vi "dlgMultiAnalysisList.vi"(7 "StandAlone (true)":bool=TRUE, 8 "error in (no error)":errorcluster) -> (0 "error out":errorcluster, 1 "Analyse":bool, 3 "FileList":string[][](array[string]))   [LabVIEW 2014]
uses:
  typedefs/eMainAction.ctl
  <vilib>/Utility/miscctls.llb/LVRowAndColumnTypeDef.ctl
  typedefs/ePathsAction.ctl
  <vilib>/Utility/file.llb/Read From Spreadsheet File (string).vi
  <vilib>/Utility/file.llb/Write To Spreadsheet File (string).vi
panel:
  in  "btnPopulate":bool
  in  "btnDelete":bool
  in  "btnClear":bool
  in  "btnInsert":bool
  in  "btnAnalyse":bool
  in  "btnCancel":bool
  in  "lstFiles":string[][](table) caption="List of Files to Analyse"
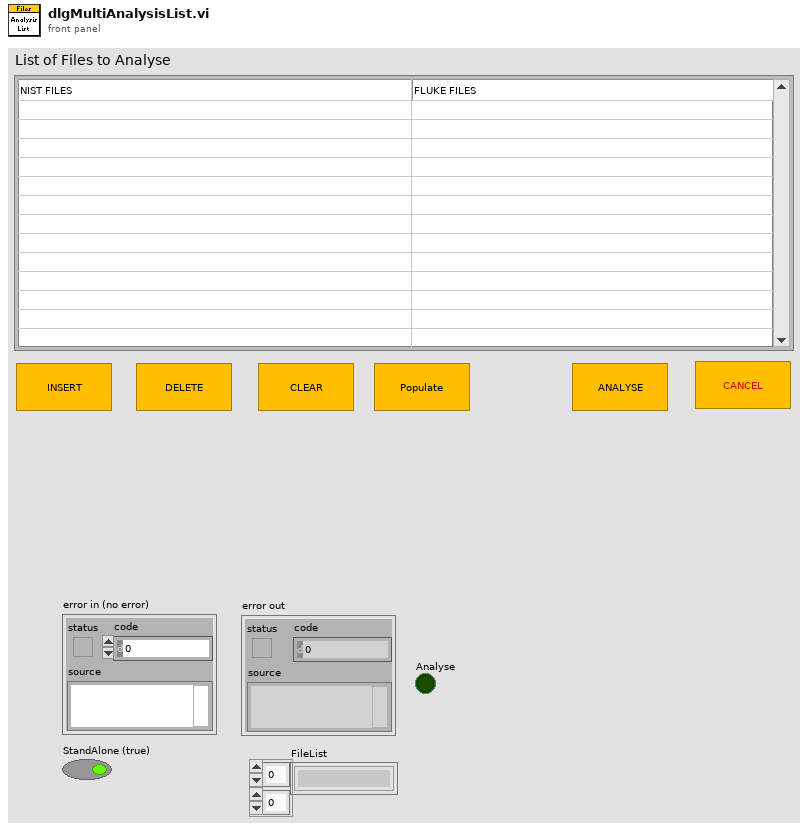
[diagram p1: front panel]
types:
  T1 = typedef "LVRowAndColumnTypeDef.ctl" = cluster{"Row":i32, "Column":i32}
  T2 = typedef "eMainAction.ctl" = enum16{"Init", "ProcessUI", "Exit"}
  T3 = typedef "ePathsAction.ctl" = enum16{"Set", "Get", "Load", "Save", "Default", "Exit"}
  T4 = typedef "Paths.ctl" = cluster{"BasePath":path, "CutPath":path, "LastCutPath":path, "CCSPath":path, "LastCCSPath":path, "ResultsPath":path}
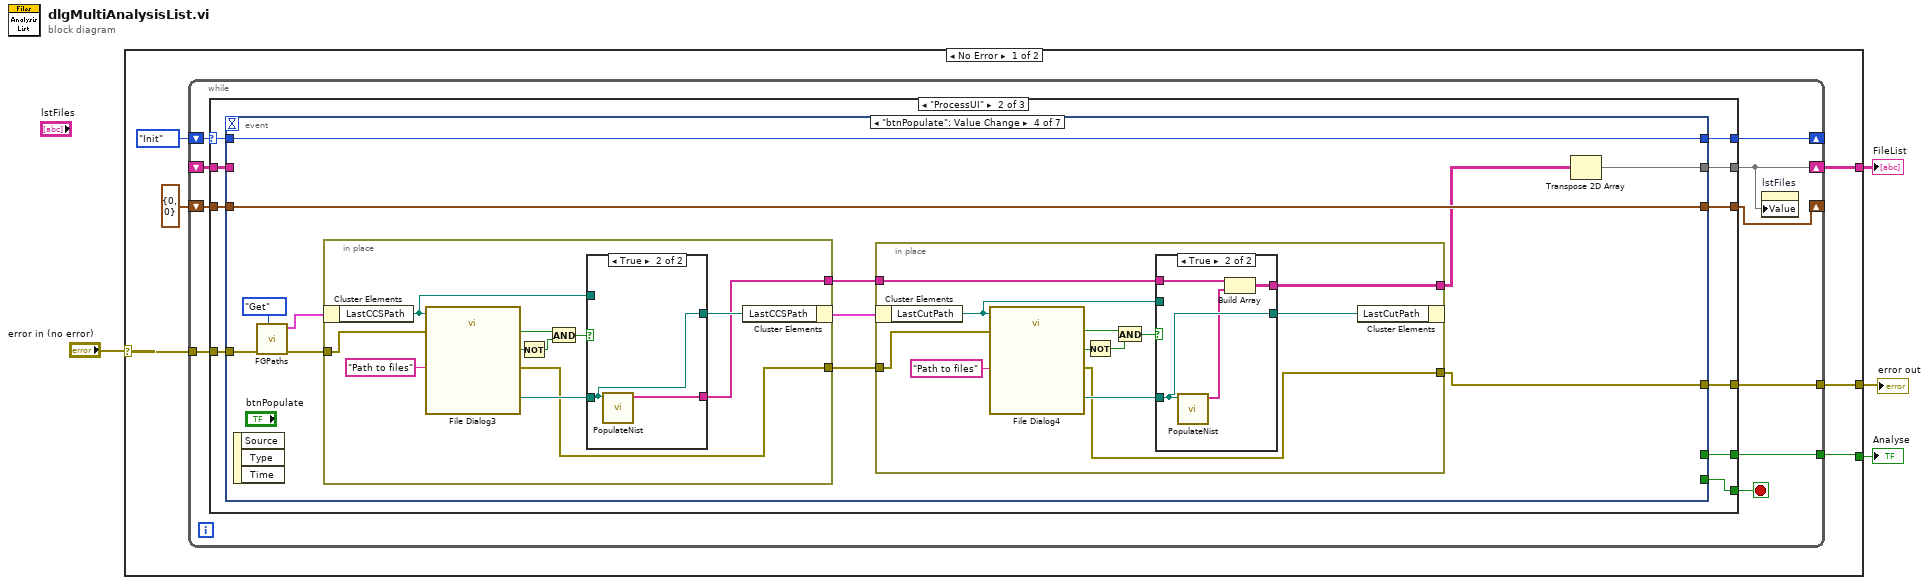
[diagram p0: block diagram]
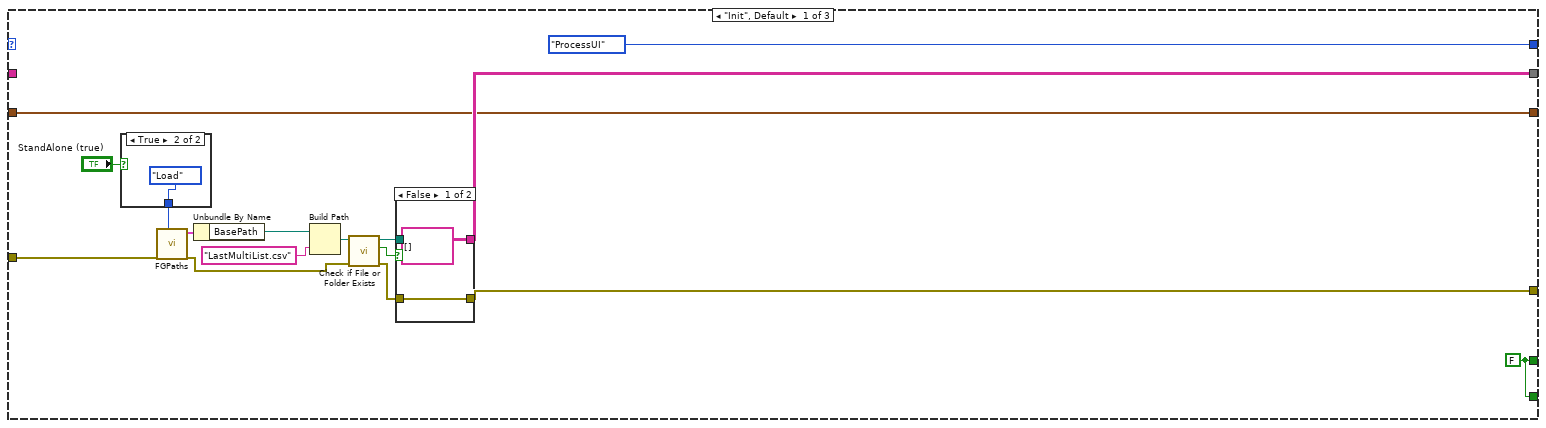
[diagram p2: hidden frame]
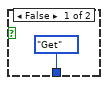
[diagram p3: hidden frame]
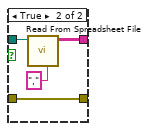
[diagram p4: hidden frame]
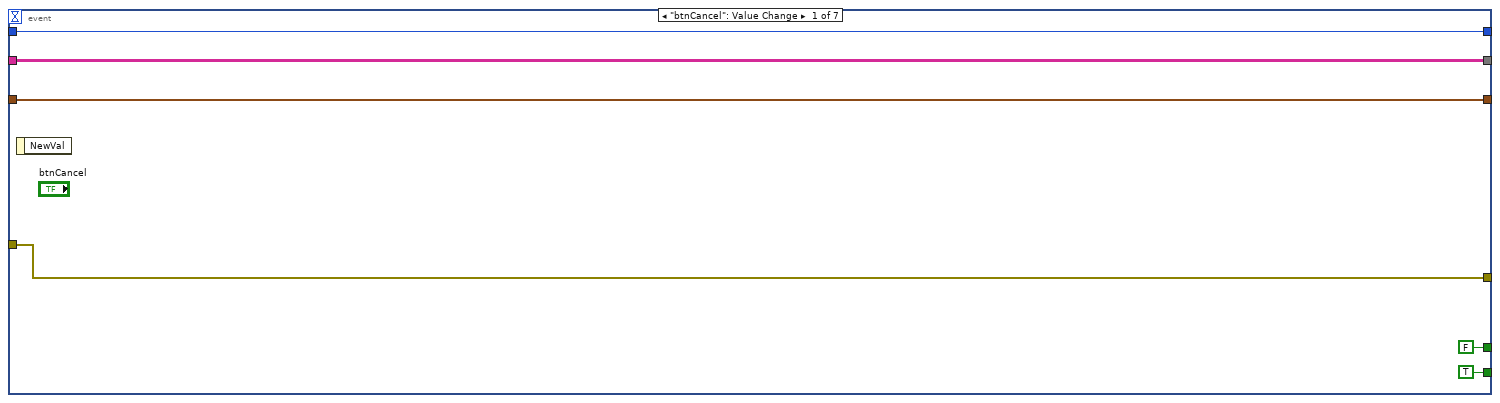
[diagram p5: hidden frame]
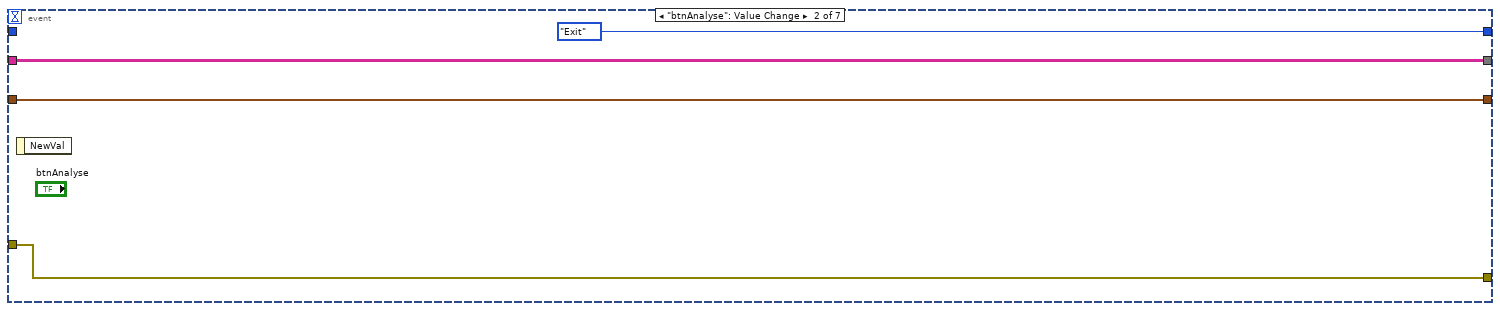
[diagram p6: hidden frame]
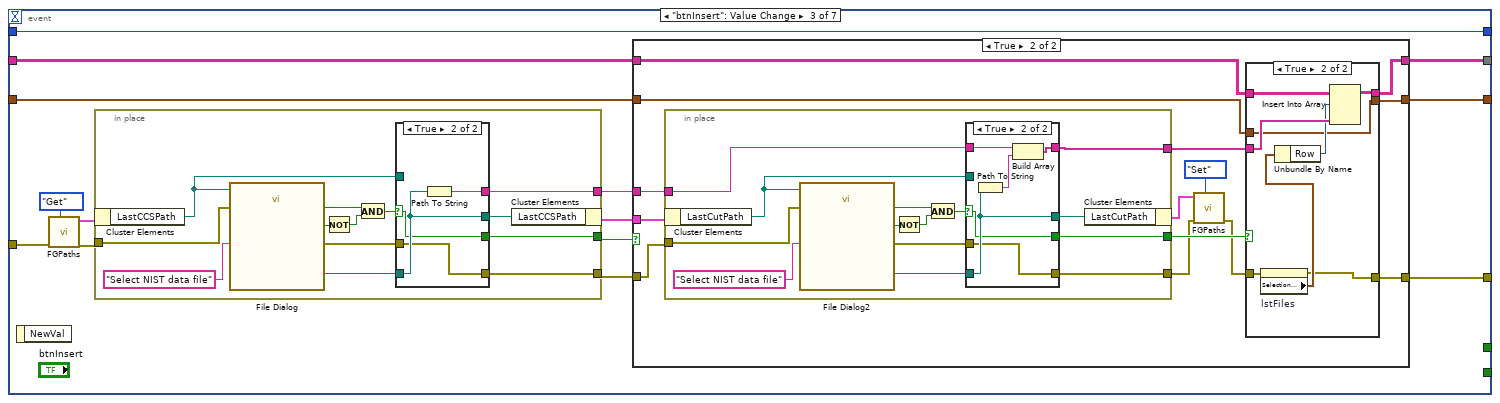
[diagram p7: hidden frame]
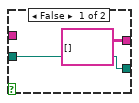
[diagram p12: hidden frame]
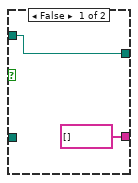
[diagram p13: hidden frame]
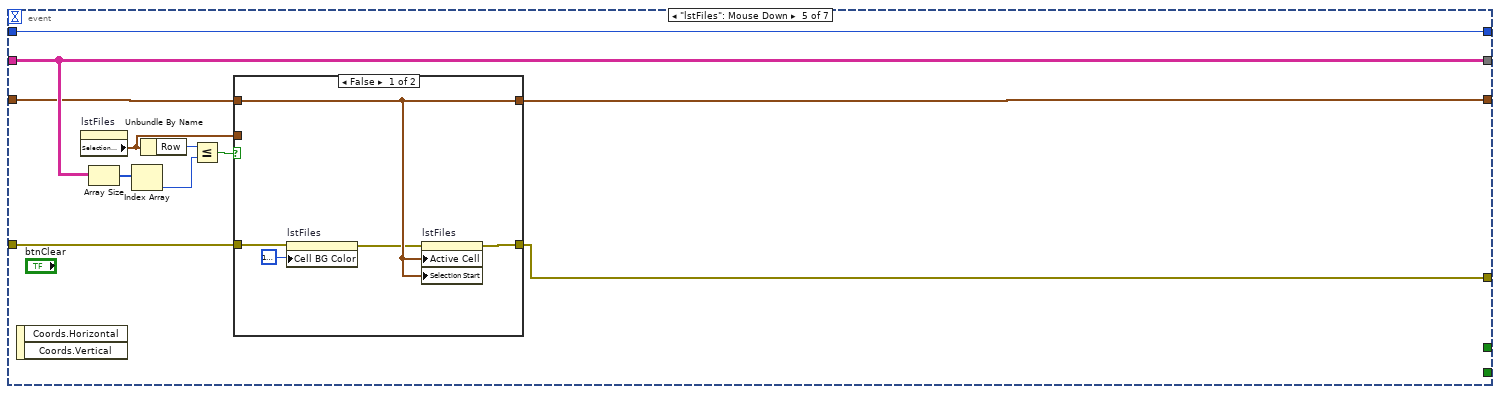
[diagram p14: hidden frame]
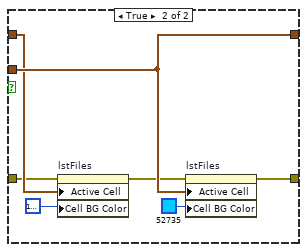
[diagram p15: hidden frame]
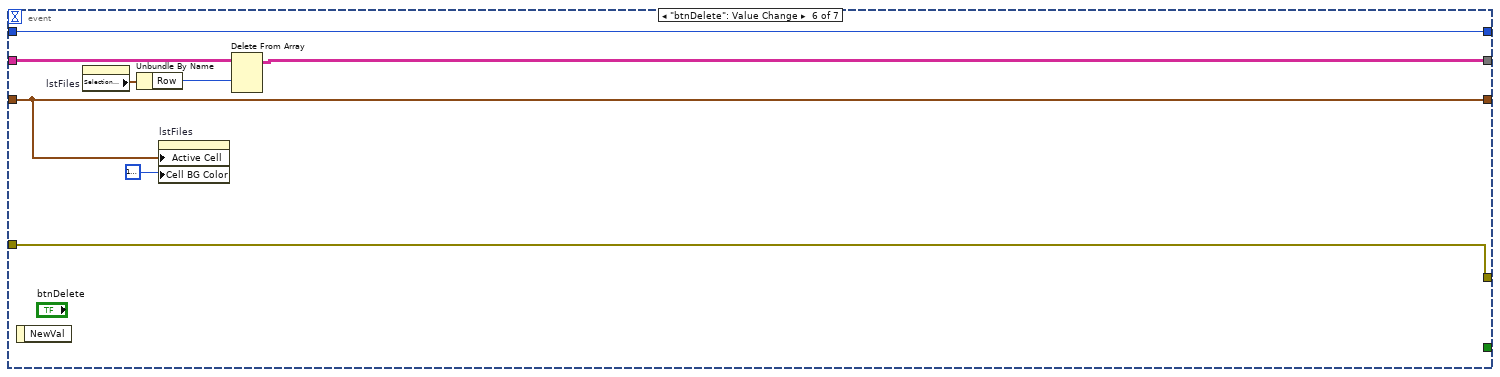
[diagram p16: hidden frame]
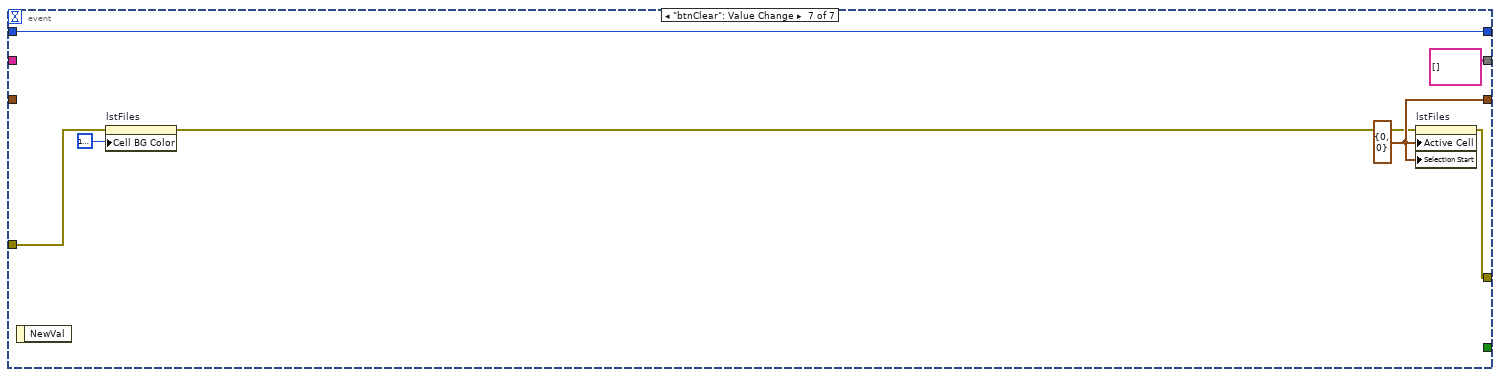
[diagram p17: hidden frame]
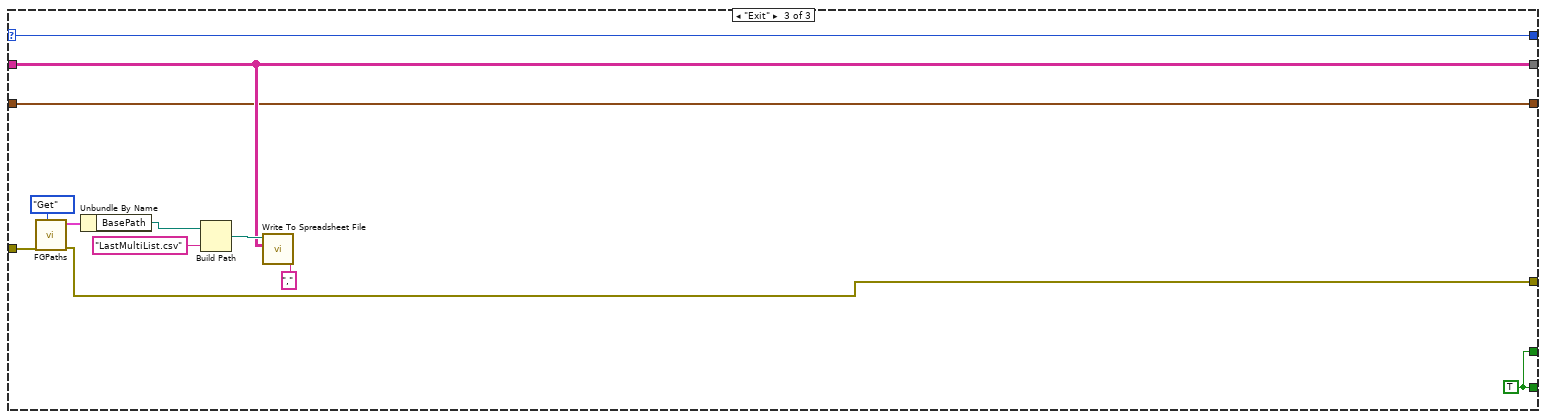
[diagram p18: hidden frame]
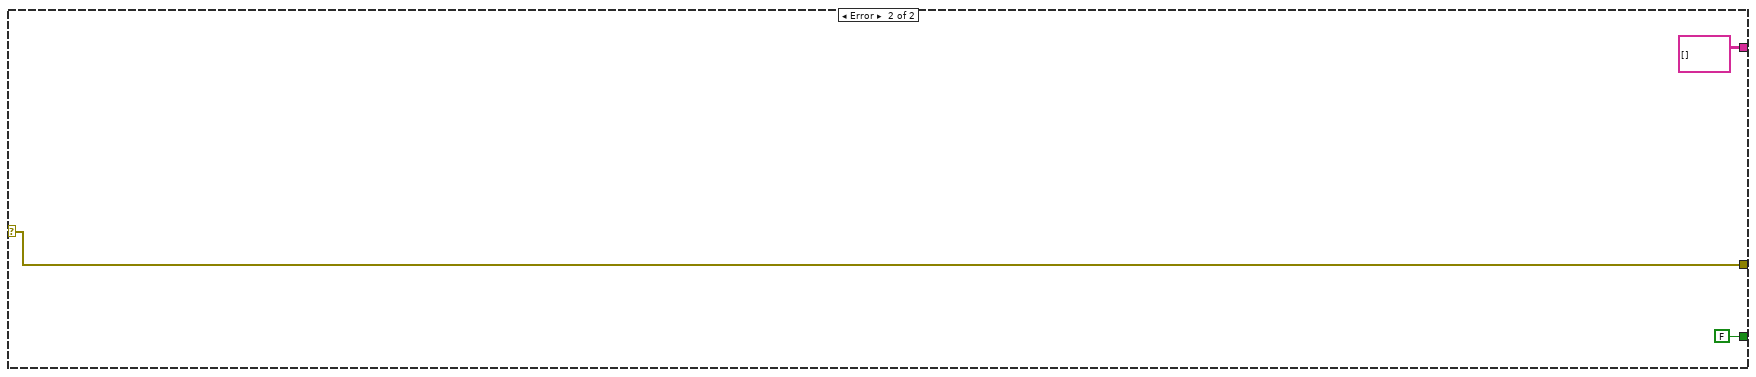
[diagram p19: hidden frame]
diagram:
  n1 = case shown="No Error" "error in (no error)" {
    selector: "error in (no error)" -> [w10 w245]
    tunnel: [w8 FALSE] -> w3
    tunnel: [w7 string[][] [] ("all rows")] -> w2
    tunnel: [w5 w245] -> w1
    frame No Error {
      n2 = while {
        tunnel: w10 -> [w20]
        shift-right: [w17] -> _
        shift-left: eMainAction."Init" ("eMainAction") -> [w19]
        shift-right: [w18] -> w7
        shift-left: _ -> [w14]
        tunnel: [w15] -> w8
        shift-right: [w13] -> _
        shift-left: T1 {"Row"=0, "Column"=0} ("Selection Start") -> [w12]
        tunnel: [w11] -> w5
        stop <- w16 stop-if-true
        n3 = case shown="\"ProcessUI\"" w19 {
          selector: w19 -> [_ w51 w235]
          tunnel: w20 -> [w26 w48 w243]
          tunnel: [w25 w50 w236] -> w18
          tunnel: [eMainAction."ProcessUI" ("eMainAction") w52 w235] -> w17
          tunnel: [w23 w54 w244] -> w16
          tunnel: [w23 w53 w244] -> w15
          tunnel: w14 -> [_ w49 w236]
          tunnel: [w22 w47 w234] -> w13
          tunnel: w12 -> [w22 w46 w234]
          tunnel: [w21 w45 w233] -> w11
          frame "Init", Default {
            w23 = FALSE
            n4 = case shown="True" "StandAlone (true)" {
              tunnel: [ePathsAction."Get" ("ePathsAction") ePathsAction."Load" ("ePathsAction")] -> w36
              frame False {
              }
              frame True {
              }
            }
            n5 = call "FGPaths.vi"("ePathsAction"=w36, "error in (no error)"=w26) -> ("error out"=w31:errorcluster, "PathsOut"=w35:T4)  [unwired: 8 in]
            n6 = Unbundle By Name(w35) -> ("BasePath"=w34:path)
            n7 = Build Path(base path=w34, name or relative path="LastMultiList.csv") -> (appended path=w32:path)
            n8 = call <vilib>:"Check if File or Folder Exists.vi"("error in (no error)"=w31, "path"=w32) -> ("error out"=w28:errorcluster, "file or folder exists?"=w29:bool, "dup path"=w30:path)  [unwired: 7 in]
            n9 = case shown="False" w29 {
              tunnel: w30 -> [_ w44]
              tunnel: w28 -> [w39 w42]
              tunnel: [w39 w42] -> w21
              tunnel: [string[][] [] ("all rows") w41] -> w25
              frame False {
              }
              frame True {
                n10 = call-poly <vilib>:"Read From Spreadsheet File.vi"("delimiter (\\t)"="," ("delimiter (\\t)"), "file path (dialog if empty)"=w44) -> ("all rows"=w41:string[][])  [unwired: 5 in, 4 out]
              }
            }
          }
          frame "ProcessUI" {
            n11 = event shown="[3] \"btnPopulate\": Value Change" {
              selector: _ -> [_ _ _ _ _ _ _]
              dyn-events: _ -> [_ _ _ _ _ _ _]
              timeout: _ -> [_ _ _ _ _ _ _]
              tunnel: [TRUE _ _ _ _ _ _] -> w54
              tunnel: [FALSE _ _ _ _ _ _] -> w53
              tunnel: [w58 eMainAction."Exit" ("eMainAction") w68 w156 w196 w220 w232] -> w52
              tunnel: w51 -> [w58 _ w68 w156 w196 w220 w232]
              tunnel: [w57 w63 w72 w155 w204 w222 string[][] [] ("all rows")] -> w50
              tunnel: w49 -> [w57 w63 w73 _ w204 w225 _]
              tunnel: w48 -> [w55 w62 w78 w161 w197 w218 w228]
              tunnel: [w56 w61 w65 w157 w199 w219 w230] -> w47
              tunnel: w46 -> [w56 w61 w66 w157 w198 w219 _]
              tunnel: [w55 w62 w67 w150 w195 w218 w226] -> w45
              event "btnCancel": Value Change {
                n12 = event-data() -> ()  [unwired: 1 in, 1 out]
              }
              event "btnAnalyse": Value Change {
                n13 = event-data() -> ()  [unwired: 1 in, 1 out]
              }
              event "btnInsert": Value Change {
                n14 = event-data() -> ()  [unwired: 1 in, 1 out]
                n15 = call "FGPaths.vi"("ePathsAction"=ePathsAction."Get", "error in (no error)"=w78) -> ("error out"=w75:errorcluster, "PathsOut"=w76:T4)  [unwired: 8 in]
                n16 = in-place {
                  in-place-border: w75 -> [w141]
                  in-place-border: [w133] -> w74
                  in-place-border: [w132] -> w69
                  in-place-border: [w130] -> w71
                  n17 = in-place-cluster #1(w76) -> ("LastCCSPath"=w136:path)
                  n18 = call "File Dialog"("start path"=w136, "prompt"="Select NIST data file", "error in"=w141) -> ("selected path"=w134:path, "exists"=w138:bool, "cancelled"=w139:bool, "error out"=w131:errorcluster)  [unwired: 9 in]
                  n19 = Not(x=w139) -> (.not. x?=w137:bool)
                  n20 = And(x=w138, y=w137) -> (x .and. y?=w140:bool)
                  n21 = case shown="True" w140 {
                    selector: w140 -> [w144 w148]
                    tunnel: w136 -> [w145 _]
                    tunnel: [w145 w149] -> w135
                    tunnel: w134 -> [_ w149]
                    tunnel: [_ w146] -> w132
                    tunnel: [w144 w148] -> w133
                    tunnel: w131 -> [w143 w147]
                    tunnel: [w143 w147] -> w130
                    frame False {
                    }
                    frame True {
                      n22 = Path To String(path=w149) -> (string=w146:string)
                    }
                  }
                  n23 = in-place-cluster #1("LastCCSPath"=w135) -> (w70:T4)
                }
                n24 = case shown="True" w74 {
                  tunnel: w73 -> [w81 w92]
                  tunnel: [w81 w91] -> w72
                  tunnel: w71 -> [w80 w94]
                  tunnel: w70 -> [_ w95]
                  tunnel: [w80 w88] -> w67
                  tunnel: w69 -> [_ w90]
                  tunnel: w66 -> [w79 w86]
                  tunnel: [w79 w87] -> w65
                  frame False {
                  }
                  frame True {
                    n25 = in-place {
                      in-place-border: w94 -> [w119]
                      in-place-border: [w111] -> w93
                      in-place-border: [w109] -> w83
                      in-place-border: w90 -> [w108]
                      in-place-border: [w107] -> w89
                      n26 = in-place-cluster #2(w95) -> ("LastCutPath"=w114:path)
                      n27 = call "File Dialog2"("start path"=w114, "prompt"="Select NIST data file", "error in"=w119) -> ("selected path"=w112:path, "exists"=w116:bool, "cancelled"=w117:bool, "error out"=w110:errorcluster)  [unwired: 9 in]
                      n28 = Not(x=w117) -> (.not. x?=w115:bool)
                      n29 = And(x=w116, y=w115) -> (x .and. y?=w118:bool)
                      n30 = case shown="True" w118 {
                        selector: w118 -> [w122 w128]
                        tunnel: w114 -> [w123 _]
                        tunnel: [w123 w129] -> w113
                        tunnel: w112 -> [_ w129]
                        tunnel: [w122 w128] -> w111
                        tunnel: w110 -> [w121 w127]
                        tunnel: [w121 w127] -> w109
                        tunnel: w108 -> [_ w125]
                        tunnel: [_ w126] -> w107
                        frame False {
                        }
                        frame True {
                          n31 = Path To String(path=w129) -> (string=w124:string)
                          n32 = Build Array(w125, w124) -> (w126:string[])
                        }
                      }
                      n33 = in-place-cluster #2("LastCutPath"=w113) -> (w85:T4)
                    }
                    n34 = call "FGPaths.vi"("ePathsAction"=ePathsAction."Set", "error in (no error)"=w83, "PathsIn"=w85) -> ("error out"=w82:errorcluster)  [unwired: 7 in, 1 out]
                    n35 = case shown="True" w93 {
                      tunnel: w92 -> [w98 w106]
                      tunnel: [w98 w105] -> w91
                      tunnel: w89 -> [_ w104]
                      tunnel: w82 -> [w97 w101]
                      tunnel: [w97 w100] -> w88
                      tunnel: [w96 w99] -> w87
                      tunnel: w86 -> [w96 w99]
                      frame False {
                      }
                      frame True {
                        n36 = property on="lstFiles" class="Tbl (strict)"(error in=w101) -> (error out=w100:errorcluster, "Selection Start"=w103:T1)  [unwired: 1 in, 1 out]
                        n37 = Unbundle By Name(w103) -> ("Row"=w102:i32)
                        n38 = Insert Into Array(array=w106, index (row)=w102, new element=w104) -> (w105:string[][])  [unwired: 1 in]
                      }
                    }
                  }
                }
              }
              event "btnPopulate": Value Change {
                n39 = event-data() -> ()  [unwired: 1 in, 3 out]
                n40 = call "FGPaths.vi"("ePathsAction"=ePathsAction."Get", "error in (no error)"=w161) -> ("error out"=w158:errorcluster, "PathsOut"=w159:T4)  [unwired: 8 in]
                n41 = in-place {
                  in-place-border: w158 -> [w189]
                  in-place-border: [w181] -> w154
                  in-place-border: [w180] -> w152
                  n42 = in-place-cluster #3(w159) -> ("LastCCSPath"=w183:path)
                  n43 = call "File Dialog3"("start path"=w183, "prompt"="Path to files", "error in"=w189) -> ("selected path"=w184:path, "exists"=w187:bool, "cancelled"=w188:bool, "error out"=w180:errorcluster)  [unwired: 9 in]
                  n44 = Not(x=w188) -> (.not. x?=w186:bool)
                  n45 = And(x=w187, y=w186) -> (x .and. y?=w185:bool)
                  n46 = case shown="True" w185 {
                    tunnel: w184 -> [_ w193]
                    tunnel: w183 -> [w192 _]
                    tunnel: [w192 w193] -> w182
                    tunnel: [string[] [] ("Array") w194] -> w181
                    frame False {
                    }
                    frame True {
                      n47 = call "PopulateNist.vi"("Path"=w193) -> ("Array"=w194:string[])  [unwired: 10 in]
                    }
                  }
                  n48 = in-place-cluster #3("LastCCSPath"=w182) -> (w153:T4)
                }
                n49 = in-place {
                  in-place-border: w154 -> [w164]
                  in-place-border: w152 -> [w172]
                  in-place-border: [w163] -> w151
                  in-place-border: [w162] -> w150
                  n50 = in-place-cluster #4(w153) -> ("LastCutPath"=w165:path)
                  n51 = call "File Dialog4"("start path"=w165, "prompt"="Path to files", "error in"=w172) -> ("selected path"=w167:path, "exists"=w169:bool, "cancelled"=w171:bool, "error out"=w162:errorcluster)  [unwired: 9 in]
                  n52 = Not(x=w171) -> (.not. x?=w170:bool)
                  n53 = And(x=w169, y=w170) -> (x .and. y?=w168:bool)
                  n54 = case shown="True" w168 {
                    tunnel: w167 -> [_ w179]
                    tunnel: [w175 w179] -> w166
                    tunnel: w165 -> [w175 _]
                    tunnel: w164 -> [_ w178]
                    tunnel: [string[][] [] w176] -> w163
                    frame False {
                    }
                    frame True {
                      n55 = call "PopulateNist.vi"("Path"=w179) -> ("Array"=w177:string[])  [unwired: 10 in]
                      n56 = Build Array(w178, w177) -> (w176:string[][])
                    }
                  }
                  n57 = in-place-cluster #4("LastCutPath"=w166) -> ()  [unwired: 1 out]
                }
                n58 = Transpose 2D Array(2D array=w151) -> (transposed array=w155:string[][])
              }
              event "lstFiles": Mouse Down {
                n59 = event-data() -> ()  [unwired: 1 in, 2 out]
                n60 = property on="lstFiles" class="Tbl (strict)"() -> ("Selection Start"=w200:T1)  [unwired: 2 in, 2 out]
                n61 = Array Size(array=w204) -> (size(s)=w203:i32[])
                n62 = Index Array(array=w203) -> (element=w202:i32)  [unwired: 1 in]
                n63 = Unbundle By Name(w200) -> ("Row"=w205:i32)
                n64 = Less Or Equal?(x=w205, y=w202) -> (x <= y?=w201:bool)
                n65 = case shown="False" w201 {
                  tunnel: w200 -> [_ w216]
                  tunnel: [w210 w216] -> w199
                  tunnel: w198 -> [w210 w215]
                  tunnel: w197 -> [w208 w213]
                  tunnel: [w206 w211] -> w195
                  frame False {
                    n66 = property on="lstFiles" class="Tbl (strict)"(error in=w208, "Cell BG Color"=u32 16777225) -> (error out=w207:errorcluster)  [unwired: 1 in, 1 out]
                    n67 = property on="lstFiles" class="Tbl (strict)"(error in=w207, "Active Cell"=w210, "Selection Start"=w210) -> (error out=w206:errorcluster)  [unwired: 1 in, 1 out]
                  }
                  frame True {
                    n68 = property on="lstFiles" class="Tbl (strict)"(error in=w213, "Active Cell"=w215, "Cell BG Color"=u32 16777225) -> (error out=w212:errorcluster)  [unwired: 1 in, 1 out]
                    n69 = property on="lstFiles" class="Tbl (strict)"(error in=w212, "Active Cell"=w216, "Cell BG Color"=u32 52735) -> (error out=w211:errorcluster)  [unwired: 1 in, 1 out]
                  }
                }
              }
              event "btnDelete": Value Change {
                n70 = event-data() -> ()  [unwired: 1 in, 1 out]
                n71 = property on="lstFiles" class="Tbl (strict)"() -> ("Selection Start"=w224:T1)  [unwired: 2 in, 2 out]
                n72 = Unbundle By Name(w224) -> ("Row"=w223:i32)
                n73 = property on="lstFiles" class="Tbl (strict)"("Active Cell"=w219, "Cell BG Color"=u32 16777225) -> ()  [unwired: 2 in, 2 out]
                n74 = Delete From Array(array=w225, index (row)=w223) -> (array with subset deleted=w222:string[][])  [unwired: 2 in, 1 out]
              }
              event "btnClear": Value Change {
                w230 = T1 {"Row"=0, "Column"=0} ("Active Cell:Active Cell")
                n75 = event-data() -> ()  [unwired: 1 in, 1 out]
                n76 = property on="lstFiles" class="Tbl (strict)"(error in=w228, "Cell BG Color"=u32 16777225) -> (error out=w227:errorcluster)  [unwired: 1 in, 1 out]
                n77 = property on="lstFiles" class="Tbl (strict)"(error in=w227, "Active Cell"=w230, "Selection Start"=w230) -> (error out=w226:errorcluster)  [unwired: 1 in, 1 out]
              }
            }
          }
          frame "Exit" {
            w244 = TRUE
            n78 = call "FGPaths.vi"("ePathsAction"=ePathsAction."Get", "error in (no error)"=w243) -> ("error out"=w233:errorcluster, "PathsOut"=w239:T4)  [unwired: 8 in]
            n79 = Unbundle By Name(w239) -> ("BasePath"=w241:path)
            n80 = Build Path(base path=w241, name or relative path="LastMultiList.csv") -> (appended path=w238:path)
            n81 = call-poly <vilib>:"Write To Spreadsheet File.vi"("delimiter (\\t)"="," ("delimiter (\\t)"), "2D data"=w236, "file path (dialog if empty)"=w238) -> ()  [unwired: 5 in, 1 out]
          }
        }
        n82 = property on="lstFiles" class="Tbl (strict)"("Value"=w18) -> ()  [unwired: 2 in, 2 out]
      }
    }
    frame Error {
    }
  }
  "error out" <- w1
  "Analyse" <- w3
  "FileList" <- w2
